vi "OOB to Logic FGV.vi"(7 "Op (Get)":enum16{"Get", "Set"}(ring), 8 "error in (no error)":errorcluster, 11 "OOB to Logic Data in":T1={"PauseResume"=FALSE, "Export"="", "ID CAN"=0, "Type CAN"=0, "DLC CAN"=0, "SEND CAN"=FALSE, "Payload CAN"=[0, 0, 0, 0, 0, 0, 0, 0, 0, 0, 0, 0, 0, 0, 0, 0, 0, 0, 0, 0, 0, 0, 0, 0, 0, 0, 0, 0, 0, 0, 0, 0, 0, 0, 0, 0, 0, 0, 0, 0, 0, 0, 0, 0, 0, 0, 0, 0, 0, 0, 0, 0, 0, 0, 0, 0, 0, 0, 0, 0, 0, 0, 0, 0], "ID LIN"=0, "DLC LIN"=0, "SEND LIN"=FALSE, "Payload LIN"=[0, 0, 0, 0, 0, 0, 0, 0], "out_str"=""} {"Payload LIN" format="%x"; "ID LIN" format="%x"; "Payload CAN" format="%x"; "Type CAN" items=["CAN Data"=0, "CAN Remote"=1, "CAN Bus Error"=2, "CAN 2.0 Data"=8, "CAN FD Data"=16, "CAN FD+BRS Data"=24, "J1939 Data"=192, "Delay"=224, "Log Trigger"=225, "Start Trigger"=226]; "ID CAN" format="%x"}) -> (0 "error out":errorcluster, 3 "OOB to Logic Data out":T1 {"Payload LIN" format="%x"; "ID LIN" format="%x"; "Payload CAN" format="%x"; "Type CAN" items=["CAN Data"=0, "CAN Remote"=1, "CAN Bus Error"=2, "CAN 2.0 Data"=8, "CAN FD Data"=16, "CAN FD+BRS Data"=24, "J1939 Data"=192, "Delay"=224, "Log Trigger"=225, "Start Trigger"=226]; "ID CAN" format="%x"})   [LabVIEW 2025, in "OOB Data Transfer.lvlib"]
uses:
  OOB Data Transfer.lvlib
  Typdefs/OOB to Logic Data.ctl
  CAN-LIN Frame Generator UI/XNET Frame Type CAN.ctl
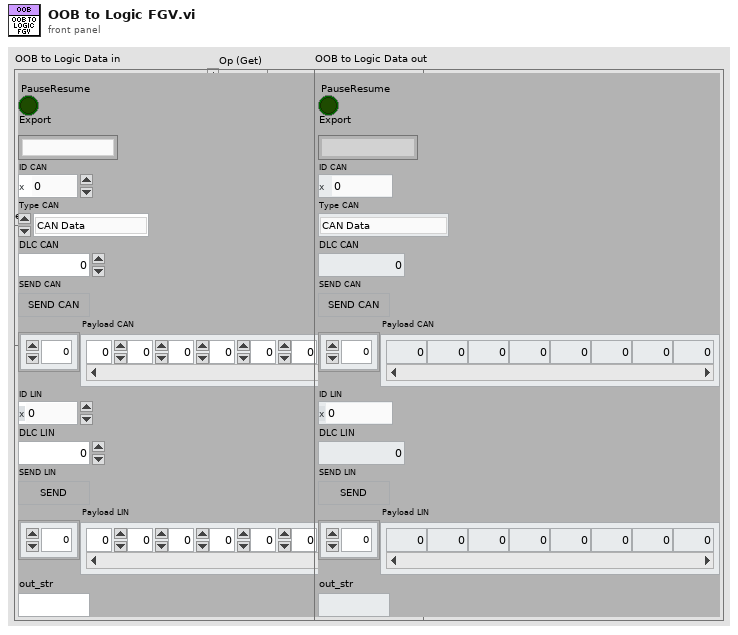
[diagram p1: front panel]
types:
  T1 = typedef "OOB Data Transfer.lvlib/OOB to Logic Data.ctl" = cluster{"PauseResume":bool, "Export":string, "ID CAN":u32, "Type CAN":T2, "DLC CAN":u32, "SEND CAN":bool, "Payload CAN":u32[], "ID LIN":u32, "DLC LIN":u32, "SEND LIN":bool, "Payload LIN":u32[], "out_str":string}
  T2 = typedef "XNET Frame Type CAN.ctl" = u32
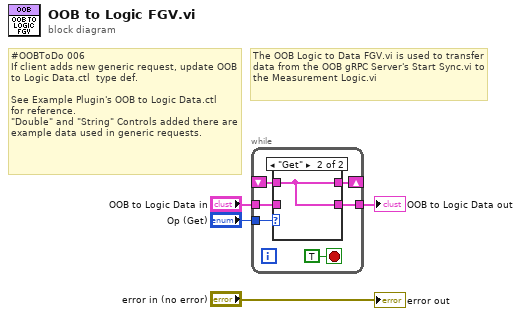
[diagram p0: block diagram]
diagram:
  # "The OOB Logic to Data FGV.vi is used to transfer data from the OOB gRPC Server's Start Sync.vi to the Measurement Logic.vi"
  # "#OOBToDo 006 \nIf client adds new generic request, update OOB to Logic Data.ctl  type def.\n \nSee Example Plugin's OOB to Logic Data.ctl for reference. \n\"Double\" and \"String\" Controls added there are example data used in generic requests."
  n1 = while {
    tunnel: "Op (Get)" -> [w9]
    tunnel: "OOB to Logic Data in" -> [w8]
    shift-right: [w7] -> _
    shift-left: _ -> [w6]
    tunnel: [w5] -> w1
    stop <- TRUE stop-if-true
    n2 = case shown="\"Get\"" w9 {
      tunnel: w8 -> [w11 _]
      tunnel: [w11 w12] -> w7
      tunnel: [w11 w12] -> w5
      tunnel: w6 -> [_ w12]
      frame "Set" {
      }
      frame "Get" {
      }
    }
  }
  "OOB to Logic Data out" <- w1
  "error out" <- "error in (no error)"
